vi "FlexWorktable Sandbox.vi"() -> ()   [LabVIEW 2017]
uses:
  Orient3d Class/Type Definitions/Quaternion.ctl
  Orient3d Class/Orient3d.lvclass
  Vec3d Class/Vec3d.lvclass
  FlexWorktable.lvclass
  Config Manager Class/Config Manager.lvclass
panel:
  out "Items out":T1
  out "Data":cluster{"X":dbl, "Y":dbl, "Z":dbl}
  out "Quaternion":T2
  out "Type":string
  in  "Regex Pattern":string=".*"
  out "Keys":string[](array[string])
  in  "Key":string
  out "error out":errorcluster
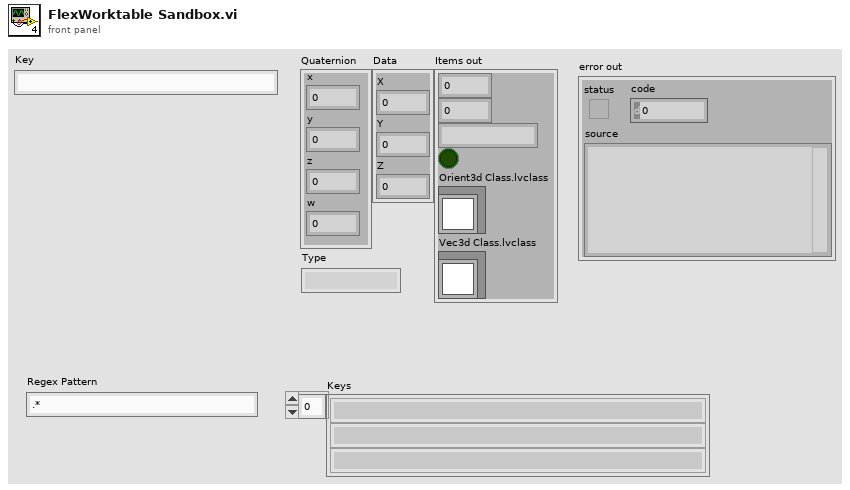
[diagram p1: front panel]
types:
  T1 = cluster{i32, dbl, string, bool, "Orient3d Class.lvclass":refnum<class "Orient3d.lvclass">, "Vec3d Class.lvclass":refnum<class "Vec3d.lvclass">}
  T2 = typedef "Quaternion.ctl" = cluster{"x":dbl, "y":dbl, "z":dbl, "w":dbl}
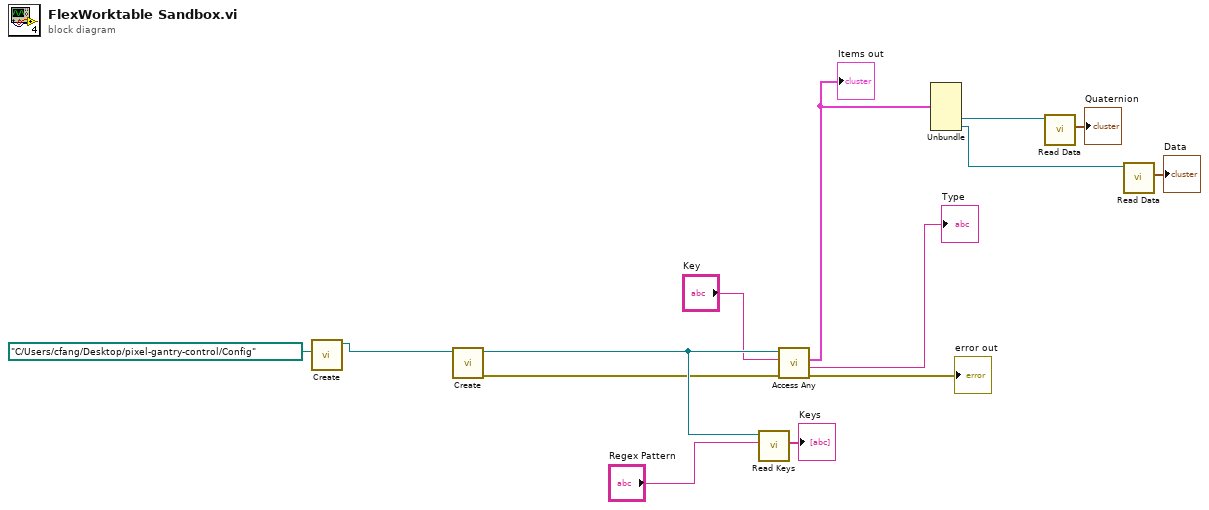
[diagram p0: block diagram]
diagram:
  n1 = call "Create.vi"("Config Root Directory"=path "C:/Users/cfang/Desktop/pixel-gantry-control/Config") -> ("Config Manager out"=w13:refnum<class "Config Manager.lvclass">)  [unwired: 9 in, 1 out]
  n2 = call "Create.vi"("Config Manager"=w13) -> ("error out"=w7:errorcluster, "FlexWorktable out"=w10:refnum<class "FlexWorktable.lvclass">)  [unwired: 9 in]
  n3 = call-dynamic "Read Keys.vi"("Selector"="Regex Pattern", "FlexWorktable in"=w10) -> ("Keys"=→"Keys":string[])  [unwired: 7 in, 2 out]
  n4 = call-dynamic "Access Any.vi"("error in (no error)"=w7, "Key"="Key", "FlexWorktable in"=w10) -> ("error out"=→"error out":errorcluster, "Type"=→"Type":string, "Items out"=w5:T1)  [unwired: 5 in, 1 out]
  "Items out" <- w5
  n5 = Unbundle(w5) -> ("Orient3d Class.lvclass"=w4:refnum<class "Orient3d.lvclass">, "Vec3d Class.lvclass"=w2:refnum<class "Vec3d.lvclass">)  [unwired: 4 out]
  n6 = call "Read Data.vi"("Orient3d in"=w4) -> ("Quaternion"=→"Quaternion":T2)  [unwired: 8 in, 2 out]
  n7 = call-dynamic "Read Data.vi"("Vec3d Class in"=w2) -> ("Data"=→"Data":cluster{"X":dbl, "Y":dbl, "Z":dbl})  [unwired: 8 in, 2 out]
